vi "Load Image From Memory (16-bit) (Core).vi"(8 "error in (no error)":errorcluster, 11 "Encoded Image":u8[](array[numeric])) -> (0 "error out":errorcluster, 2 "Image (16-bit)":T1)   [LabVIEW 2020, in "G-Image.lvlib"]
doc: "Load an image file from a byte array."
uses:
  G-Image.lvlib
  lib/g_image_32.dll
  Controls/Image 16-bit.ctl
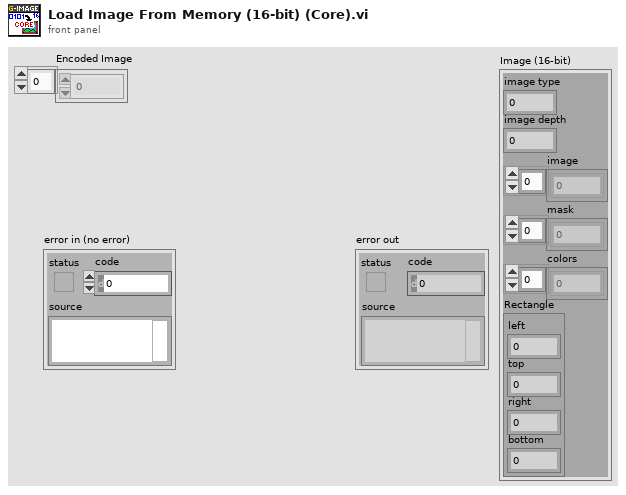
[diagram p1: front panel]
types:
  T1 = typedef "G-Image.lvlib/Image 16-bit.ctl" = cluster{"image type":i32, "image depth":i32, "image":u16[], "mask":u8[], "colors":u32[], "Rectangle":cluster{"left":i16, "top":i16, "right":i16, "bottom":i16}}
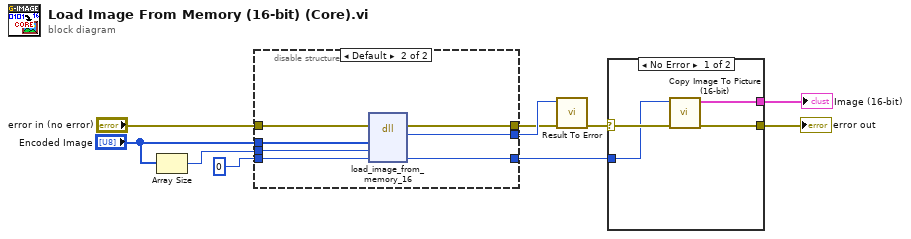
[diagram p0: block diagram]
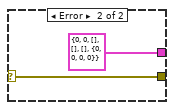
[diagram p2: hidden frame]
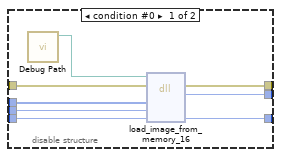
[diagram p3: hidden frame]
diagram:
  n1 = Array Size(array="Encoded Image") -> (size(s)=w2:i32)
  n2 = disable-structure shown="Default" {
    disable-tunnel: [w17 w25] -> w7
    disable-tunnel: "error in (no error)" -> [w16 w24]
    disable-tunnel: "Encoded Image" -> [w15 w23]
    disable-tunnel: [w14 w22] -> w8
    disable-tunnel: [w13 w20] -> w4
    disable-tunnel: i64 0 ("count") -> [w12 w21]
    disable-tunnel: w2 -> [w11 w19]
    frame condition #0 {
      n3 = call "Debug Path.vi"() -> ("Debug Path"=w18:path)  [unwired: 11 in]
      n4 = dll-call lib="?" fn="load_image_from_memory_16"(path in=w18, error in=w16, "encoded_image"=w15, "encoded_image_size"=w11, "image_out"=w12) -> (error out=w17:errorcluster, "result"=w14:i32, "image_out"=w13:i64)  [unwired: 3 in, 1 out]
    }
    frame condition #1 (active) {
      n5 = dll-call lib="C:/github/dataflowg/g-image/src/LabVIEW/G-Image/lib/g_image_*.*" fn="load_image_from_memory_16"(error in=w24, "encoded_image"=w23, "encoded_image_count"=w19, "image_out"=w21) -> (error out=w25:errorcluster, "result"=w22:i32, "image_out"=w20:i64)  [unwired: 4 in, 1 out]
    }
  }
  n6 = call "Result To Error.vi"("error in (no error)"=w7, "Result Code"=w8) -> ("error out"=w6:errorcluster)  [unwired: 9 in]
  n7 = case shown="No Error" w6 {
    selector: w6 -> [w29 w31]
    tunnel: [w27 w31] -> w10
    tunnel: w4 -> [w28 _]
    tunnel: [w26 T1 {"image type"=0, "image depth"=0, "image"=[], "mask"=[], "colors"=[], "Rectangle"={"left"=0, "top"=0, "right"=0, "bottom"=0}} ("Image (16-bit)")] -> w1
    frame No Error {
      n8 = call "Copy Image To Picture (16-bit).vi"("error in (no error)"=w29, "image_ptr"=w28) -> ("error out"=w27:errorcluster, "Image (16-bit)"=w26:T1)  [unwired: 8 in]
    }
    frame Error {
    }
  }
  "error out" <- w10
  "Image (16-bit)" <- w1
